vi "Configure Multiple Tone.vi"(0 "VISA resource name":refnum<visa-resource-name>, 1 "Enable Multiple Tones (T:Enable)":bool=TRUE, 5 "Initialize Phase (0: Fixed)":u16(ring) items=["Fixed", "Random"], 7 "Random Seed (0: Fixed)":u16(ring) items=["Fixed", "Random"], 9 "Frequency Spacing (10 kHz)":dbl=10000.0, 11 "error in (no error)":errorcluster, 12 "Number Of Tones (8)":i32=8, 13 "Alignment (1: Center)":u16(ring)=1 items=["Left", "Center", "Right"]) -> (4 "VISA resource name out":refnum<visa-resource-name>, 15 "error out":errorcluster)   [LabVIEW 2011, in "Agilent PSG MXG Series.lvlib"]
doc: "Initializes the phase for the multitone waveform, assigns the frequency spacing and defines the number of tones.\n\n<B>Notes:</B>\n(1) This VI is valid only in E8267C, E8267D, N5182A.\n\n(2) For E8267C, this VI is valid only when the instrument installs <B>Option 002</B> (Internal baseband generator) or <B>Option 602</B> (Digital bus baseband generator).\n\n(3) For E8267D, this VI is valid only when the instrument installs <B>Option 601</B> or <B>Option 602</B> (Internal baseband generator).\n\n(4) For N5182A, this VI is valid only when the instrument installs <B>Option 651</B> or <B>Option 652</B> or <B>Option 654</B> (Internal baseband generator), and <B>Option 430</B> (Multitone and two-tone)."
uses:
  Agilent PSG MXG Series.lvlib
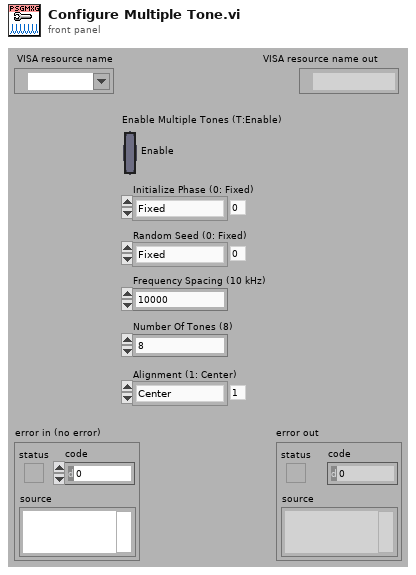
[diagram p1: front panel]
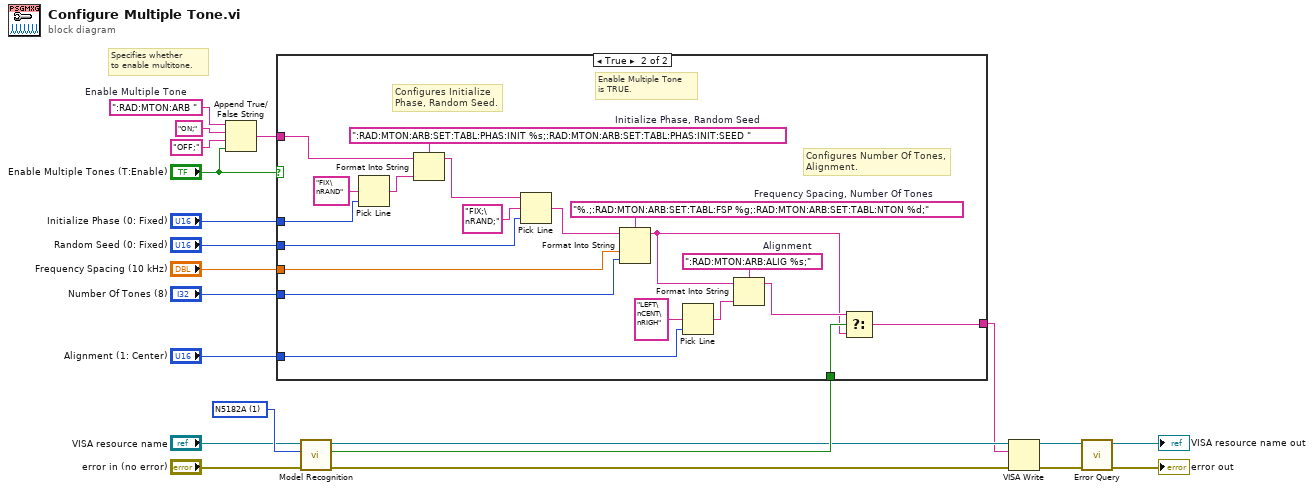
[diagram p0: block diagram]
diagram:
  w12 = u16 1 items=["N5181A"=0, "N5182A"=1, "E8241A"=5, "E8244A"=6, "E8251A"=7, "E8254A"=8, "E8247C"=10, "E8257C"=11, "E8267C"=12, "E8257D"=15, "E8267D"=16] ("Model Type (0: N5181A)")
  w21 = ":RAD:MTON:ARB "  # Enable Multiple Tone
  # "Specifies whether\nto enable multitone."
  n1 = Append True/False String(1:"Enable Multiple Tones (T:Enable)", 2:"OFF;" ("false string"), 3:"ON;" ("true string"), 4:w21) -> (0:w18:string)
  n2 = call "Model Recognition.vi"("error in (no error)"="error in (no error)", "Model Type (0: N5181A)"=w12, "VISA resource name"="VISA resource name") -> ("error out"=w9:errorcluster, "Is Model Correct"=w11:bool, "VISA resource name out"=w10:refnum<visa-resource-name>)  [unwired: 6 in]
  n3 = case shown="True" "Enable Multiple Tones (T:Enable)" {
    tunnel: w18 -> [w22 w42]
    tunnel: "Initialize Phase (0: Fixed)" -> [_ w38]
    tunnel: "Random Seed (0: Fixed)" -> [_ w35]
    tunnel: "Frequency Spacing (10 kHz)" -> [_ w32]
    tunnel: "Number Of Tones (8)" -> [_ w31]
    tunnel: "Alignment (1: Center)" -> [_ w27]
    tunnel: w11 -> [_ w26]
    tunnel: [w22 w23] -> w8
    frame False {
      # "Enable Multiple Tone\nis FALSE."
    }
    frame True {
      w30 = ":RAD:MTON:ARB:ALIG %s;"  # Alignment
      w33 = "%.;:RAD:MTON:ARB:SET:TABL:FSP %g;:RAD:MTON:ARB:SET:TABL:NTON %d;"  # Frequency Spacing, Number Of Tones
      w41 = ":RAD:MTON:ARB:SET:TABL:PHAS:INIT %s;:RAD:MTON:ARB:SET:TABL:PHAS:INIT:SEED "  # Initialize Phase, Random Seed
      # "Enable Multiple Tone\nis TRUE."
      # "Configures Number Of Tones,\nAlignment."
      # "Configures Initialize\nPhase, Random Seed."
      n4 = Pick Line(multi-line string="FIX\nRAND", line index=w38) -> (output string=w40:string)  [unwired: 1 in]
      n5 = Format Into String(format string=w41, initial string=w42, w40) -> (resulting string=w37:string)  [unwired: 1 in, 1 out]
      n6 = Pick Line(string ("")=w37, multi-line string="FIX;\nRAND;", line index=w35) -> (output string=w34:string)
      n7 = Format Into String(format string=w33, initial string=w34, w32, w31) -> (resulting string=w24:string)  [unwired: 1 in, 1 out]
      n8 = Pick Line(multi-line string="LEFT\nCENT\nRIGH", line index=w27) -> (output string=w29:string)  [unwired: 1 in]
      n9 = Format Into String(format string=w30, initial string=w24, w29) -> (resulting string=w25:string)  [unwired: 1 in, 1 out]
      n10 = Select(t=w25, s=w26, f=w24) -> (s? t:f=w23:string)
    }
  }
  n11 = VISA Write(VISA resource name=w10, write buffer=w8, error in (no error)=w9) -> (VISA resource name out=w7:refnum<visa-resource-name>, error out=w6:errorcluster)  [unwired: 1 out]
  n12 = call "Error Query.vi"("error in (no error)"=w6, "VISA resource name"=w7) -> ("error out"=→"error out":errorcluster, "VISA resource name out"=→"VISA resource name out":refnum<visa-resource-name>)  [unwired: 6 in, 2 out]
